vi "equipment.vi"() -> ()   [LabVIEW 2016]
uses:
  <vilib>/Platform/TimedLoop/XDataNode/timing_clust.ctl
  <vilib>/Platform/TimedLoop/XDataNode/nitl_modes.ctl
  <vilib>/Platform/TimedLoop/XDataNode/wakeup.ctl
  <instrlib>/Lake Shore 425/Public/Data/Field Data (Single Reading).vi
  <vilib>/platform/TimedLoop/XDataNode/XDataNode.xnode
  <instrlib>/Lake Shore 425/Lake Shore 425.lvlib
  <vilib>/Platform/TimedLoop/XDataNode/XDNodeRunTimeDep.lvlib
panel:
  out "XY Graph":cluster{"X":dbl, "Y":dbl}[](graph)
  in  "Period (ms)":i64
  out "Error":errorcluster
  in  "stop":bool
  out "Waveform Chart":dbl[](graph)
  out "error out 3":errorcluster
  out "error out 2":errorcluster
  out "error out 1":errorcluster
  out "Probe Sensitivity 3":dbl=0.001 format="%^.3e"
  out "Probe Serial Number 3":string
  out "Probe Type  3":u16(ring)=40 items=["High Sensitivity"=40, "High Stability"=41, "Ultra-High Sensitivity"=42, "User Programmable Cable / High Sensitivity Probe"=50, "User Programmable Cable / High Stability Probe"=51, "User Programmable Cable / Ultra-High Sensitivity Probe"=52]
  out "Probe Sensitivity 2":dbl=0.001 format="%^.3e"
  out "Probe Serial Number 2":string
  out "Probe Type  2":u16(ring)=40 items=["High Sensitivity"=40, "High Stability"=41, "Ultra-High Sensitivity"=42, "User Programmable Cable / High Sensitivity Probe"=50, "User Programmable Cable / High Stability Probe"=51, "User Programmable Cable / Ultra-High Sensitivity Probe"=52]
  out "Probe Sensitivity":dbl=0.001 format="%^.3e"
  out "Probe Serial Number":string
  out "Probe Type":u16(ring)=40 items=["High Sensitivity"=40, "High Stability"=41, "Ultra-High Sensitivity"=42, "User Programmable Cable / High Sensitivity Probe"=50, "User Programmable Cable / High Stability Probe"=51, "User Programmable Cable / Ultra-High Sensitivity Probe"=52]
  in  "VISA Gaussmeter 3":refnum<visa-resource-name>
  in  "VISA Gaussmeter 2":refnum<visa-resource-name>
  in  "VISA Gaussmeter 1":refnum<visa-resource-name>
  in  "Gaussmeter 3":bool
  in  "Gaussmeter 2":bool
  in  "Gaussmeter 1":bool
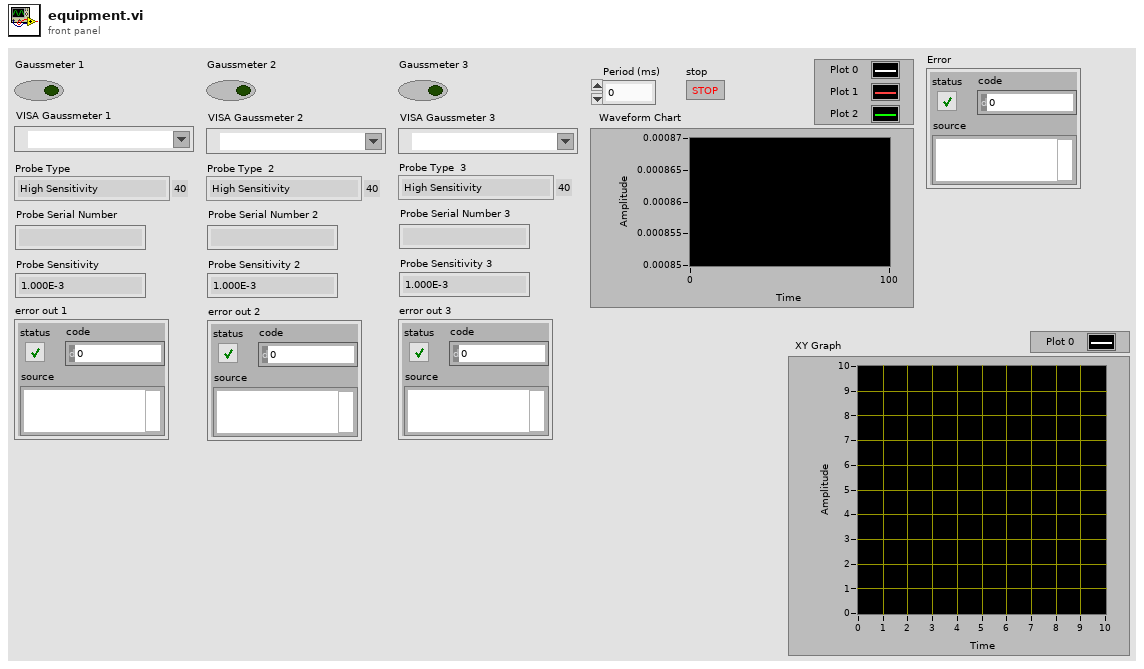
[diagram p1: front panel]
types:
  T1 = typedef "XDNodeRunTimeDep.lvlib/timing_clust.ctl" = cluster{"Expected End [f-1]":u64, "Actual End [f-1]":u64, "Finished Late? [f-1]":bool, "Expected End [i-1]":u64, "Actual End [i-1]":u64, "Finished Late? [i-1]":bool, "Expected Start [i]":u64, "Actual Start [i]":u64, "Expected Start [f]":u64, "Actual Start [f]":u64, "Source Name":string, "Structure Name":string, "Period":i64, "Deadline":i64, "Offset":i64, "Start":i64, "Priority":i32, "Timeout":i32, "Mode":T2, "Wakeup Reason":T3, "Error":errorcluster, "Source Type":string, "Secondary Source Type":string, "Global End Time":u64, "Global Start Time":u64, "Frame Duration":u64, "Iteration Duration":u64, "Assigned CPU":i32, "I/O Scan Engine Mode":u32}
  T2 = typedef "XDNodeRunTimeDep.lvlib/nitl_modes.ctl" = enum32{"No Change", "Process missed periods, maintain original phase", "Discard missed periods, maintain original phase", "Process missed periods, ignore original phase", "Discard missed periods, ignore original phase"}
  T3 = typedef "XDNodeRunTimeDep.lvlib/wakeup.ctl" = enum32{"Normal", "Aborted", "Asynchronous wakeup", "Timing source error", "Timed loop error", "Timeout"}
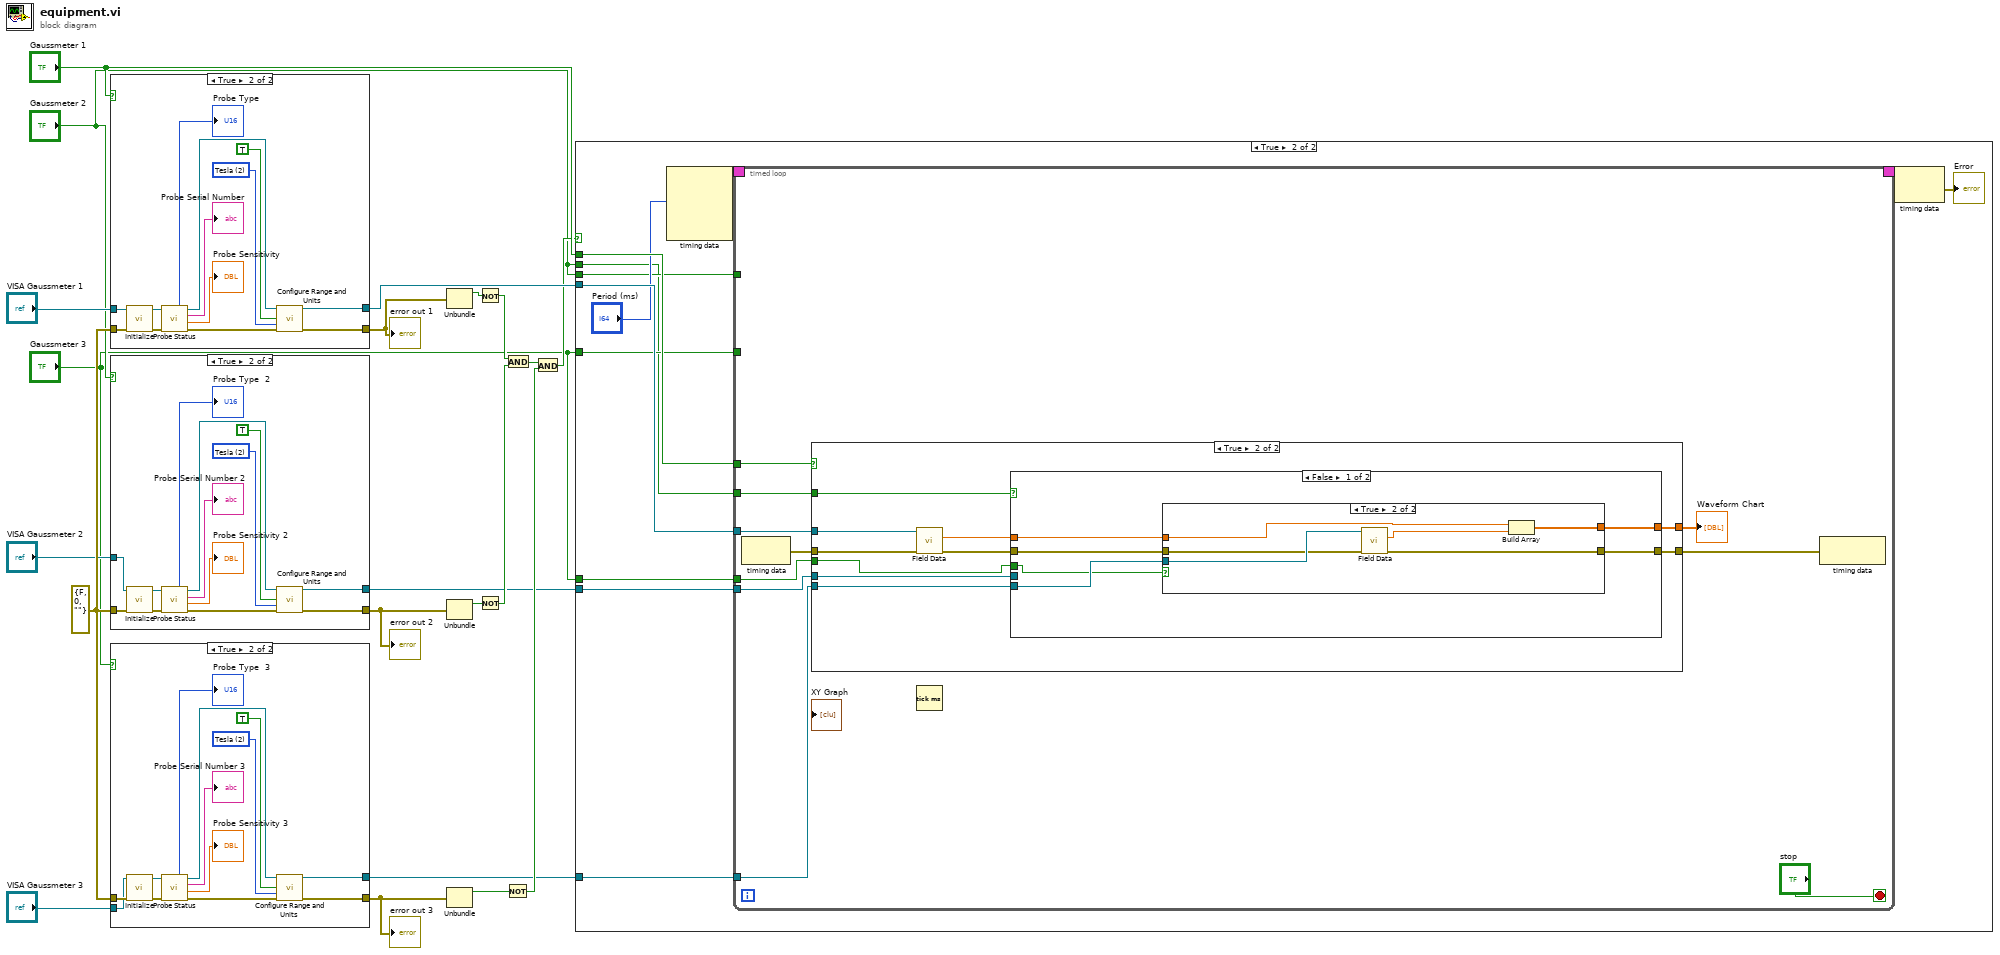
[diagram p0: block diagram]
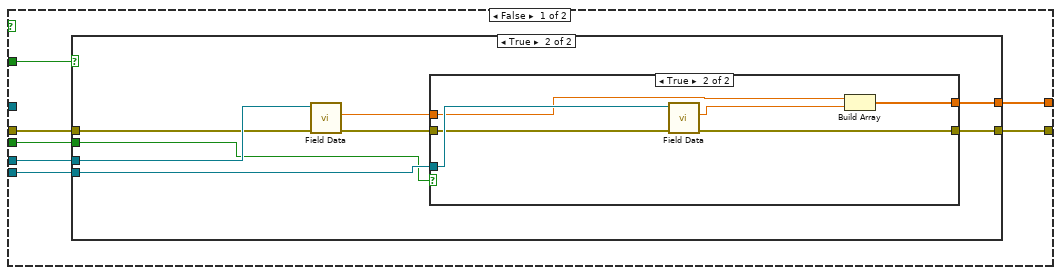
[diagram p3: hidden frame]
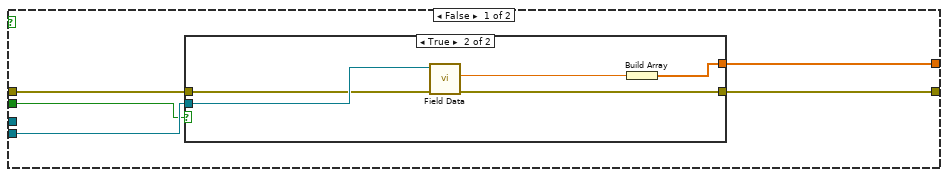
[diagram p4: hidden frame]
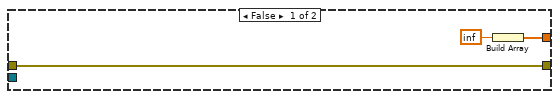
[diagram p5: hidden frame]
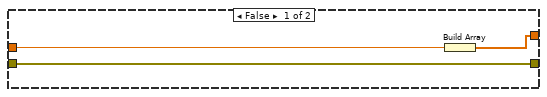
[diagram p6: hidden frame]
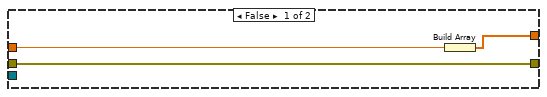
[diagram p7: hidden frame]
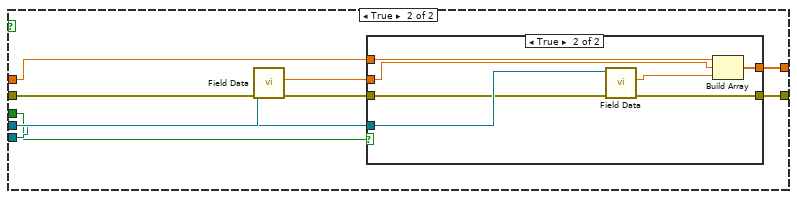
[diagram p8: hidden frame]
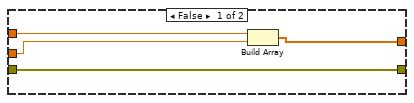
[diagram p9: hidden frame]
diagram:
  w21 = errorcluster {"status"=FALSE, "code"=0, "source"=""} ("error out")
  n1 = case shown="True" "Gaussmeter 1" {
    tunnel: [w23 w28] -> w15
    tunnel: w21 -> [w23 w36]
    tunnel: [w22 w25] -> w19
    tunnel: "VISA Gaussmeter 1" -> [w22 w24]
    frame False {
    }
    frame True {
      w26 = u16 2 items=["Gauss"=1, "Tesla"=2, "Oersted"=3, "Amp/meter"=4] ("Field Units (1:Gauss)")
      n2 = call <instrlib>:"Initialize.vi"("error in (no error)"=w36, "VISA resource name"=w24) -> ("error out"=w34:errorcluster, "VISA resource name out"=w35:refnum<visa-resource-name>)  [unwired: 8 in]
      n3 = call <instrlib>:"Probe Status.vi"("error in (no error)"=w34, "VISA resource name"=w35) -> ("error out"=w29:errorcluster, "Probe Sensitivity"=→"Probe Sensitivity":dbl, "Probe Serial Number"=→"Probe Serial Number":string, "VISA resource name out"=w30:refnum<visa-resource-name>, "Probe Type"=→"Probe Type":u16)  [unwired: 4 in, 1 out]
      n4 = call <instrlib>:"Configure Range and Units.vi"("VISA resource name"=w30, "Auto Range (F: Off)"=TRUE, "Field Units (1:Gauss)"=w26, "error in (no error)"=w29) -> ("VISA resource name out"=w25:refnum<visa-resource-name>, "error out"=w28:errorcluster)  [unwired: 10 in]
    }
  }
  "error out 1" <- w15
  n5 = case shown="True" "Gaussmeter 2" {
    tunnel: w21 -> [w38 w51]
    tunnel: [w38 w41] -> w14
    tunnel: "VISA Gaussmeter 2" -> [w37 w40]
    tunnel: [w37 w39] -> w3
    frame False {
    }
    frame True {
      w50 = u16 2 items=["Gauss"=1, "Tesla"=2, "Oersted"=3, "Amp/meter"=4] ("Field Units (1:Gauss)")
      n6 = call <instrlib>:"Initialize.vi"("error in (no error)"=w51, "VISA resource name"=w40) -> ("error out"=w42:errorcluster, "VISA resource name out"=w43:refnum<visa-resource-name>)  [unwired: 8 in]
      n7 = call <instrlib>:"Probe Status.vi"("error in (no error)"=w42, "VISA resource name"=w43) -> ("error out"=w48:errorcluster, "Probe Sensitivity"=→"Probe Sensitivity 2":dbl, "Probe Serial Number"=→"Probe Serial Number 2":string, "VISA resource name out"=w47:refnum<visa-resource-name>, "Probe Type"=→"Probe Type  2":u16)  [unwired: 4 in, 1 out]
      n8 = call <instrlib>:"Configure Range and Units.vi"("VISA resource name"=w47, "Auto Range (F: Off)"=TRUE, "Field Units (1:Gauss)"=w50, "error in (no error)"=w48) -> ("VISA resource name out"=w39:refnum<visa-resource-name>, "error out"=w41:errorcluster)  [unwired: 10 in]
    }
  }
  "error out 2" <- w14
  n9 = case shown="True" "Gaussmeter 3" {
    tunnel: w21 -> [w53 w66]
    tunnel: [w53 w58] -> w13
    tunnel: "VISA Gaussmeter 3" -> [w52 w55]
    tunnel: [w52 w54] -> w4
    frame False {
    }
    frame True {
      w65 = u16 2 items=["Gauss"=1, "Tesla"=2, "Oersted"=3, "Amp/meter"=4] ("Field Units (1:Gauss)")
      n10 = call <instrlib>:"Initialize.vi"("error in (no error)"=w66, "VISA resource name"=w55) -> ("error out"=w57:errorcluster, "VISA resource name out"=w56:refnum<visa-resource-name>)  [unwired: 8 in]
      n11 = call <instrlib>:"Probe Status.vi"("error in (no error)"=w57, "VISA resource name"=w56) -> ("error out"=w63:errorcluster, "Probe Sensitivity"=→"Probe Sensitivity 3":dbl, "Probe Serial Number"=→"Probe Serial Number 3":string, "VISA resource name out"=w62:refnum<visa-resource-name>, "Probe Type"=→"Probe Type  3":u16)  [unwired: 4 in, 1 out]
      n12 = call <instrlib>:"Configure Range and Units.vi"("VISA resource name"=w62, "Auto Range (F: Off)"=TRUE, "Field Units (1:Gauss)"=w65, "error in (no error)"=w63) -> ("VISA resource name out"=w54:refnum<visa-resource-name>, "error out"=w58:errorcluster)  [unwired: 10 in]
    }
  }
  "error out 3" <- w13
  n13 = Unbundle(w15) -> ("status"=w10:bool)  [unwired: 2 out]
  n14 = Unbundle(w14) -> ("status"=w8:bool)  [unwired: 2 out]
  n15 = Unbundle(w13) -> ("status"=w6:bool)  [unwired: 2 out]
  n16 = Not(x=w10) -> (.not. x?=w9:bool)
  n17 = Not(x=w8) -> (.not. x?=w7:bool)
  n18 = Not(x=w6) -> (.not. x?=w5:bool)
  n19 = And(x=w9, y=w7) -> (x .and. y?=w12:bool)
  n20 = And(x=w12, y=w5) -> (x .and. y?=w11:bool)
  n21 = case shown="True" w11 {
    tunnel: "Gaussmeter 1" -> [_ w76]
    tunnel: w19 -> [_ w74]
    tunnel: w4 -> [_ w72]
    tunnel: w3 -> [_ w71]
    tunnel: "Gaussmeter 3" -> [_ w70]
    tunnel: "Gaussmeter 2" -> [_ w69]
    tunnel: "Gaussmeter 2" -> [_ w68]
    tunnel: "Gaussmeter 3" -> [_ w67]
    frame False {
    }
    frame True {
      n22 = node-c288("Period (ms)") -> (w78:T1)  [unwired: 3 in]
      n23 = timed-loop {
        timing: w78 -> [_]
        timing-out: [_] -> w77
        tunnel: w76 -> [w88]
        tunnel: w74 -> [w86]
        tunnel: w72 -> [w83]
        tunnel: w71 -> [w82]
        tunnel: w70 -> [_]
        tunnel: w69 -> [_]
        tunnel: w68 -> [w81]
        tunnel: w67 -> [w80]
        stop <- "stop" stop-if-true
        n24 = node-c288() -> (w84:errorcluster)  [unwired: 1 in]
        n25 = case shown="True" w88 {
          tunnel: w86 -> [_ w135]
          tunnel: [w89 w130] -> w85
          tunnel: w84 -> [w94 w134]
          tunnel: w83 -> [w92 w133]
          tunnel: w82 -> [w91 w132]
          tunnel: w81 -> [w95 w128]
          tunnel: w80 -> [w93 w127]
          tunnel: [w90 w126] -> w79
          frame False {
            n26 = case shown="True" w95 {
              tunnel: w91 -> [_ w116]
              tunnel: [w96 w112] -> w89
              tunnel: w94 -> [w100 w115]
              tunnel: w92 -> [w99 w114]
              tunnel: [w97 w110] -> w90
              tunnel: w93 -> [w98 w109]
              frame False {
                n27 = case shown="True" w98 {
                  tunnel: w99 -> [_ w108]
                  tunnel: [w103 w107] -> w96
                  tunnel: w100 -> [w103 w106]
                  tunnel: [w102 w105] -> w97
                  frame False {
                    n28 = Build Array(inf) -> (w102:dbl[])
                  }
                  frame True {
                    n29 = call-poly <instrlib>:"Field Data.vi"("error in (no error)"=w106, "VISA resource name"=w108) -> ("error out"=w107:errorcluster, "Field Reading"=w104:dbl)  [unwired: 7 in, 1 out]
                    n30 = Build Array(w104) -> (w105:dbl[])
                  }
                }
              }
              frame True {
                n31 = call-poly <instrlib>:"Field Data.vi"("error in (no error)"=w115, "VISA resource name"=w116) -> ("error out"=w113:errorcluster, "Field Reading"=w111:dbl)  [unwired: 7 in, 1 out]
                n32 = case shown="True" w109 {
                  tunnel: w114 -> [_ w125]
                  tunnel: [w119 w124] -> w112
                  tunnel: w113 -> [w119 w123]
                  tunnel: w111 -> [w118 w121]
                  tunnel: [w117 w120] -> w110
                  frame False {
                    n33 = Build Array(w118) -> (w117:dbl[])
                  }
                  frame True {
                    n34 = call-poly <instrlib>:"Field Data.vi"("error in (no error)"=w123, "VISA resource name"=w125) -> ("error out"=w124:errorcluster, "Field Reading"=w122:dbl)  [unwired: 7 in, 1 out]
                    n35 = Build Array(w121, w122) -> (w120:dbl[])
                  }
                }
              }
            }
          }
          frame True {
            n36 = call-poly <instrlib>:"Field Data.vi"("error in (no error)"=w134, "VISA resource name"=w135) -> ("error out"=w131:errorcluster, "Field Reading"=w129:dbl)  [unwired: 7 in, 1 out]
            n37 = case shown="False" w128 {
              tunnel: w132 -> [_ w159]
              tunnel: [w136 w155] -> w130
              tunnel: w131 -> [w140 w158]
              tunnel: w133 -> [w139 w157]
              tunnel: w129 -> [w141 w153]
              tunnel: [w137 w152] -> w126
              tunnel: w127 -> [w138 w151]
              frame False {
                n38 = case shown="True" w138 {
                  tunnel: w139 -> [_ w150]
                  tunnel: [w144 w149] -> w136
                  tunnel: w140 -> [w144 w148]
                  tunnel: w141 -> [w143 w147]
                  tunnel: [w142 w146] -> w137
                  frame False {
                    n39 = Build Array(w143) -> (w142:dbl[])
                  }
                  frame True {
                    n40 = call-poly <instrlib>:"Field Data.vi"("error in (no error)"=w148, "VISA resource name"=w150) -> ("error out"=w149:errorcluster, "Field Reading"=w145:dbl)  [unwired: 7 in, 1 out]
                    n41 = Build Array(w147, w145) -> (w146:dbl[])
                  }
                }
              }
              frame True {
                n42 = call-poly <instrlib>:"Field Data.vi"("error in (no error)"=w158, "VISA resource name"=w159) -> ("error out"=w156:errorcluster, "Field Reading"=w154:dbl)  [unwired: 7 in, 1 out]
                n43 = case shown="True" w151 {
                  tunnel: w157 -> [_ w170]
                  tunnel: [w163 w169] -> w155
                  tunnel: w156 -> [w163 w168]
                  tunnel: w154 -> [w161 w166]
                  tunnel: w153 -> [w162 w165]
                  tunnel: [w160 w164] -> w152
                  frame False {
                    n44 = Build Array(w162, w161) -> (w160:dbl[])
                  }
                  frame True {
                    n45 = call-poly <instrlib>:"Field Data.vi"("error in (no error)"=w168, "VISA resource name"=w170) -> ("error out"=w169:errorcluster, "Field Reading"=w167:dbl)  [unwired: 7 in, 1 out]
                    n46 = Build Array(w165, w166, w167) -> (w164:dbl[])
                  }
                }
              }
            }
          }
        }
        "Waveform Chart" <- w79
        n47 = Tick Count (ms)() -> ()  [unwired: 1 out]
        n48 = node-c288(w85) -> ()  [unwired: 1 out]
      }
      n49 = node-c288(w77) -> (→"Error":errorcluster)
    }
  }
